vi "niFpgaRegisterPaletteMethodNodeMergeVi.vi"   [LabVIEW 2017]
doc: "Invokes a method on a register item on the FPGA."
uses:
  <vilib>/rvi/DataTransferAndStorage/Container/XNode/niFpgaContainer.xnode
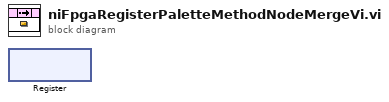
[diagram p0: block diagram]
diagram:
  n1 = xnode "Register"() -> ()  [unwired: 1 in, 1 out]
